vi "Doppler gating v2.vi"() -> ()   [LabVIEW 2022 SP3]
doc: "I. Description:\nThis example demonstrates how to use the timed loop to efficiently acquire a continuous amount of data (Waveform) using the DAQ devices internal clock and a counter to execute the timed loop only when all the data is available to Read.\n\nII. Instructions for Running:\n1. Select the physical channel to correspond to where your signal is input on the DAQ device. \n2. Enter the Source of Events. In this case we want the loop to execute on each AI sample clock pulse.\n3. Enter the counter you want to use to measure the events. In this example ctr0 is used as the default.\n4. Enter the minimum and maximum voltages.\nNote: For better accuracy try to match the input range to the expected voltage level of the measured signal.\n5. Select the number of samples to Read. Note: Because of the way this example uses the timed loop this parameter cannot be changed on-the-fly. \n6. Set the rate of the acquisition\nNote: The rate should be AT LEAST twice as fast as the maximum frequency component of the signal being acquired.\n\nIII. Block Diagram Steps:\n1. Create an Analog Input voltage channel.\n2. Set the timing type of the analog input task to Sample Clock. \n3. Call the DAQmx Create Timing Source (Digital Edge Counter) VI and specify the edge count to be the Samples to Read. What this does is cause the timed loop to only fire once it has received \"samples to read\" number of edges from the AI sample clock. This is an efficient use of CPU resources because the loop, and therefore the AI Read, will only execute once all of the samples are available.\n4. Call the Start VI to start the acquisition.\n5. Read the waveform once all the samples to read are available. In this approach the Read VI behaves in a \"non-blocking\" fashion, since it does not have to wait for samples to become available.\n6. Call the Clear Task VI to Clear the Task.\n7. Use the popup dialog box to display an error if any.\n\nIV. I/O Connections Overview:\nMake sure your signal input terminal matches the Physical Channel I/O Control. For further connection information, refer to your hardware reference manual."
uses:
  <vilib>/Utility/error.llb/DialogType.ctl
  <vilib>/DAQmx/read.llb/DAQmx Read.vi
  <vilib>/DAQmx/create/channels.llb/DAQmx Create Virtual Channel.vi
  <vilib>/DAQmx/configure/timing.llb/DAQmx Timing.vi
  <vilib>/DAQmx/miscellaneous.llb/DAQmx Fill In Error Info.vi
  Instance          12 25Saved   Doppler gating v2 .vi
  Instance          14 25Saved   Doppler gating v2 .vi
  <vilib>/gmath/NI_Gmath.lvlib
panel:
  out "Intensity Chart":dbl[][](graph)
  out "Waveform Chart":waveform(dbl)[](graph)=[{"t0"=timestamp(3271083278.6561875 s since 1904-01-01), "dt"=6.25e-05, "Y"=array[5000 elements], "attributes"=variant("NI_ChannelName"=variant(string "Dev1/ai0"), "NI_UnitDescription"=variant(string "Volts"))}]
  in  "window length":i32=5000 caption="Samples to Read"
  in  "time increment":i32=100 caption="Samples to Read"
  in  "Samples to Read":i32=5000
  in  "Physical Channel":tag="Dev1/ai0"
  in  "Minimum Value":dbl=-10.0 format="%0.2f"
  in  "Maximum Value":dbl=10.0 format="%0.2f"
  in  "stop":bool
  in  "Sample Rate":dbl=16000.0 caption="Sample Rate (Hz)" format="%0.2f"
  # "For instructions, select Help>>Show Context Help"
  # "Channel Parameters"
  # "Timing Parameters"
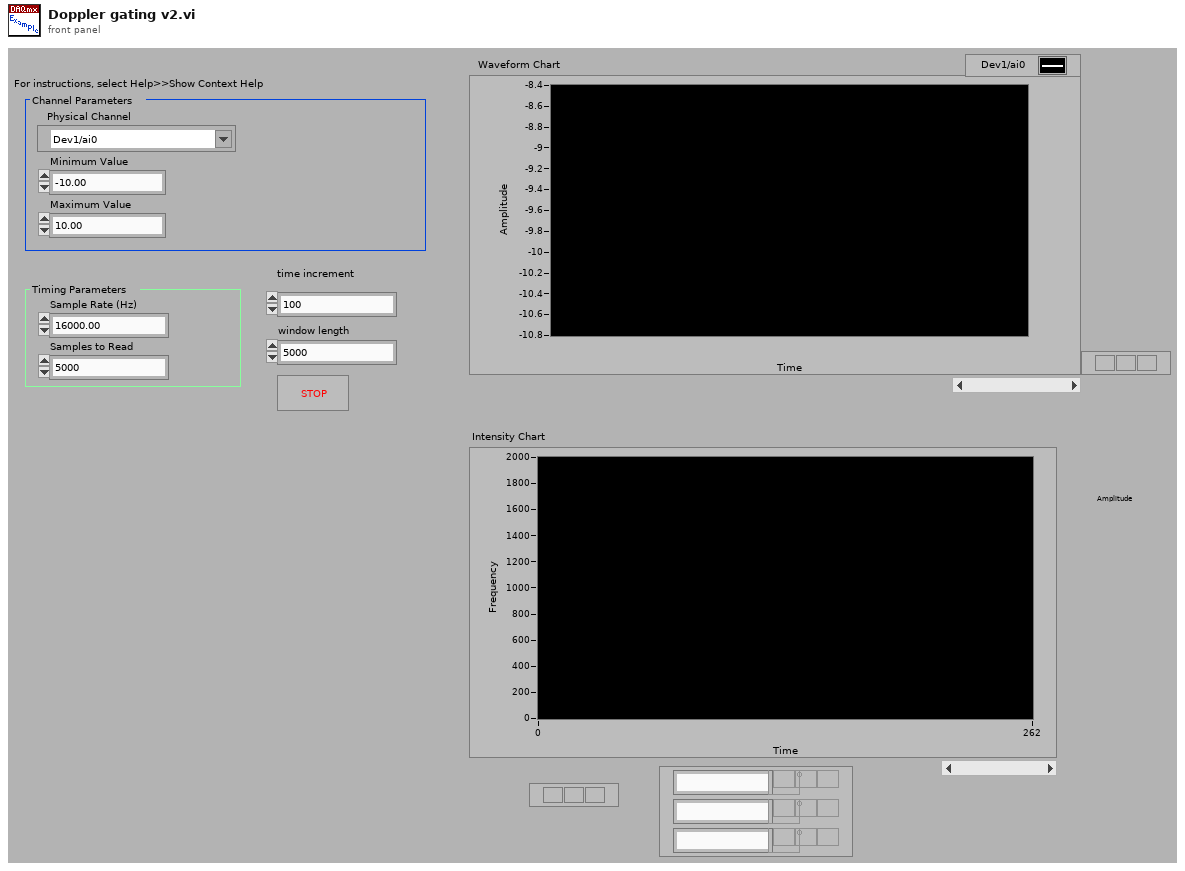
[diagram p1: front panel]
types:
  T1 = typedef "DialogType.ctl" = u16
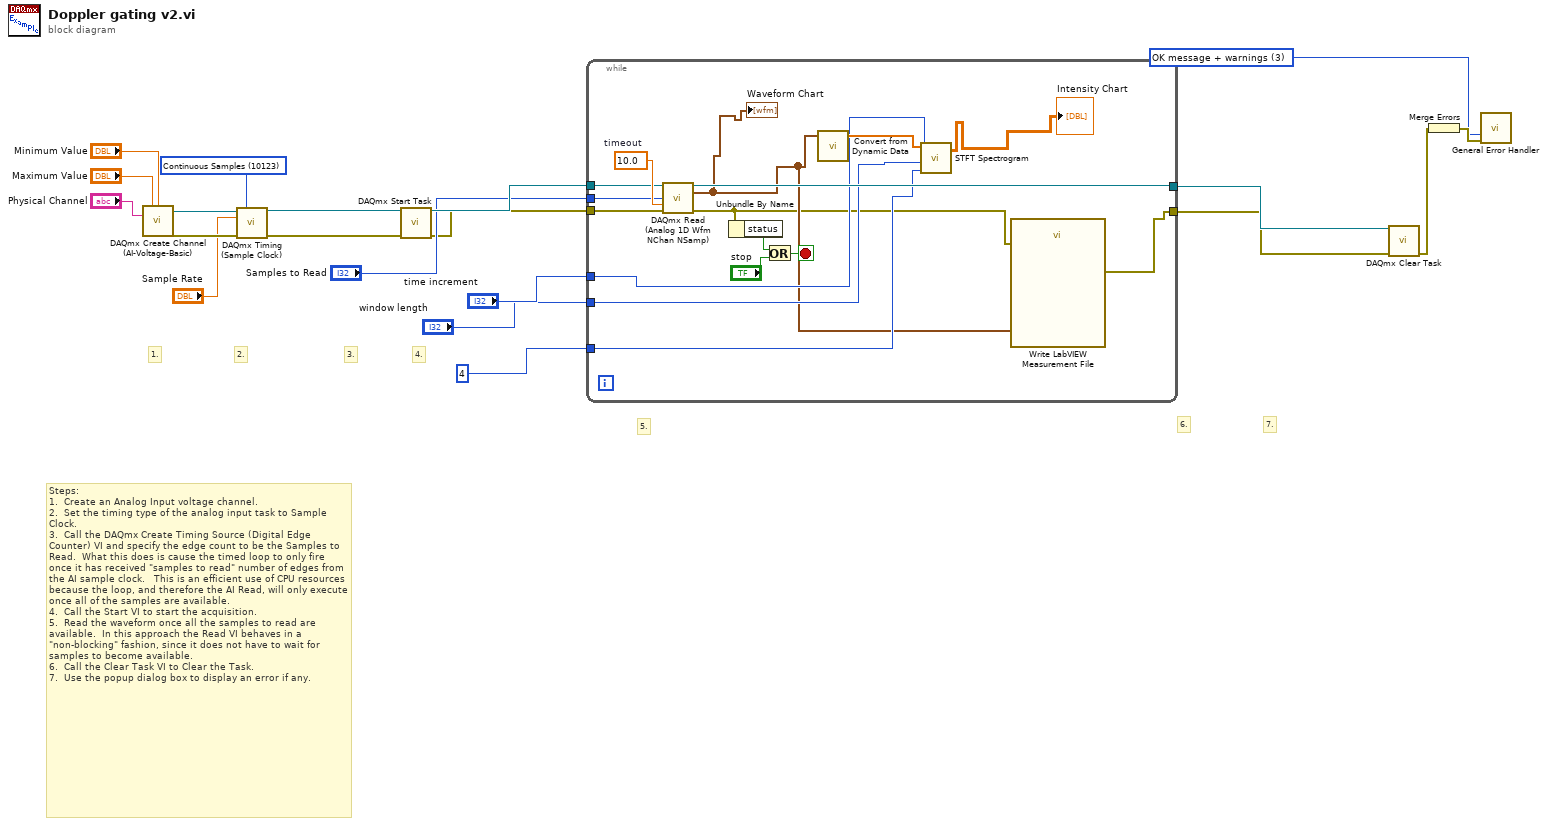
[diagram p0: block diagram]
diagram:
  w5 = T1 3 items=["no dialog", "OK message", "continue or stop message", "OK message + warnings", "continue/stop + warnings"] ("type of dialog (OK msg:1)")
  w14 = 10123 items=["Finite Samples"=10178, "Continuous Samples"=10123] ("sample mode")
  # "7."
  # "6."
  # "5."
  # "4."
  # "3."
  # "Steps:\n1.  Create an Analog Input voltage channel.\n2.  Set the timing type of the analog input task to Sample Clock. \n3.  Call the DAQmx Create Timing Source (Digital Edge Counter) VI and specify the edge count to be the Samples to Read.  What this does is cause the timed loop to only fire once it has received \"samples to read\" number of edges from the AI sample clock.   This is an efficient use of CPU resources because the loop, and therefore the AI Read, will only execute once all of the samples are available.\n4.  Call the Start VI to start the acquisition.\n5.  Read the waveform once all the samples to read are available.  In this approach the Read VI behaves in a \"non-blocking\" fashion, since it does not have to wait for samples to become available.\n6.  Call the Clear Task VI to Clear the Task.\n7.  Use the popup dialog box to display an error if any."
  # "1."
  # "2."
  n1 = call-poly <vilib>:"DAQmx Create Channel (AI-Voltage-Basic).vi"("maximum value"="Maximum Value", "minimum value"="Minimum Value", "physical channels"="Physical Channel") -> ("task out"=w17:refnum<k21>, "error out"=w18:errorcluster)  [unwired: 6 in, 5 out]
  n2 = call-poly <vilib>:"DAQmx Timing (Sample Clock).vi"("task/channels in"=w17, "sample mode"=w14, "rate"="Sample Rate", "error in"=w18) -> ("task out"=w11:refnum<k21>, "error out"=w1:errorcluster)  [unwired: 3 in, 7 out]
  n3 = call <vilib>:"DAQmx Start Task.vi"("task/channels in"=w11, "error in"=w1) -> ("task out"=w10:refnum<k21>, "error out"=w8:errorcluster)  [unwired: 12 out]
  n4 = while {
    tunnel: [w36] -> w16
    tunnel: [w21] -> w13
    tunnel: w8 -> [w31]
    tunnel: w10 -> [w30]
    tunnel: "Samples to Read" -> [w29]
    tunnel: "time increment" -> [w25]
    tunnel: "window length" -> [w28]
    tunnel: 4 -> [w27]
    stop <- w34 stop-if-true
    w32 = 10.0  # timeout
    n5 = call-poly <vilib>:"DAQmx Read (Analog 1D Wfm NChan NSamp).vi"("task/channels in"=w30, "number of samples per channel"=w29, "timeout"=w32, "error in"=w31) -> ("task out"=w36:refnum<k21>, "data"=w23:waveform(dbl)[], "error out"=w22:errorcluster)  [unwired: 9 out]
    "Waveform Chart" <- w23
    n6 = Unbundle By Name(w22) -> ("status"=w35:bool)
    n7 = Or(x=w35, y="stop") -> (x .or. y?=w34:bool)
    n8 = call "Convert from Dynamic Data"("Dynamic Data Type"=w23) -> ("Array"=w26:dbl[])  [unwired: 3 out]
    n9 = call <vilib>:"STFT Spectrogram.vi"("window selector"=w27, "window length"=w28, "time increment"=w25, "X"=w26) -> ("STFT Spectrogram {X}"=→"Intensity Chart":dbl[][])  [unwired: 1 out]
    n10 = call "Write LabVIEW Measurement File"("error in (no error)"=w22, "Signals"=w23) -> ("error out"=w21:errorcluster)  [unwired: 4 in, 5 out]
  }
  n11 = call <vilib>:"DAQmx Clear Task.vi"("task in"=w16, "error in"=w13) -> ("error out"=w7:errorcluster)  [unwired: 13 out]
  n12 = Merge Errors(w7) -> (w6:errorcluster)
  n13 = call <vilib>:"General Error Handler.vi"("type of dialog (OK msg:1)"=w5, "error in (no error)"=w6) -> ()  [unwired: 1 in, 13 out]
